vi "String.Remove Invalide Characters from File Name.vi"(8 "error in":errorcluster, 11 "File Name":string) -> (0 "error out":errorcluster, 3 "Valid File Name":string)   [LabVIEW 2018]
panel:
  # "Invalid file name characters for Windows:"
  # "A filename cannot contain any of the following characters:\n  \\ / : * ? \" < > |"
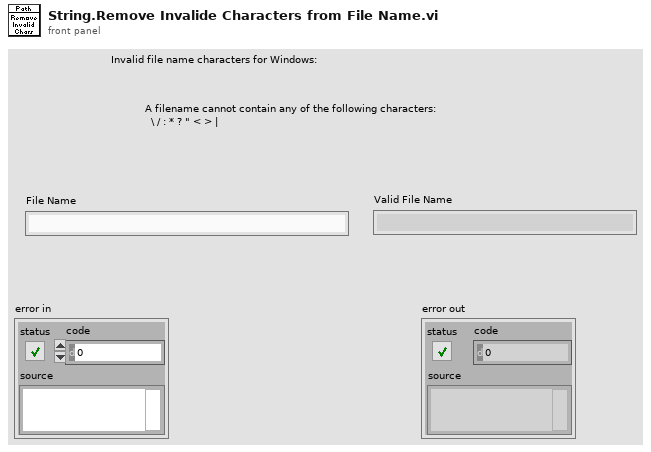
[diagram p1: front panel]
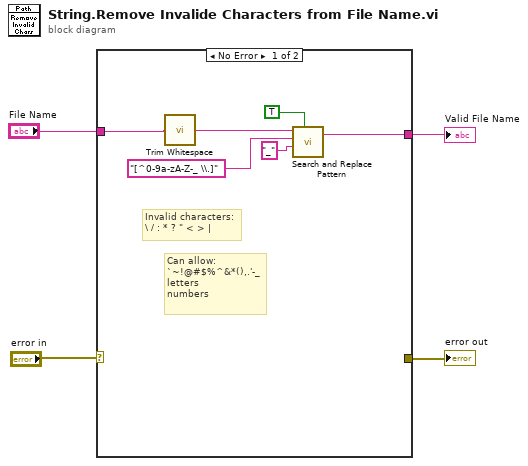
[diagram p0: block diagram]
diagram:
  n1 = case shown="No Error" "error in" {
    selector: "error in" -> [_ w11]
    tunnel: [w7 w12] -> w4
    tunnel: "File Name" -> [w6 w12]
    tunnel: [_ w11] -> w1
    frame No Error {
      # "Can allow:\n`~!@#$%^&*(),.'-_\nletters\nnumbers"
      # "Invalid characters:\n\\ / : * ? \" < > |"
      n2 = call <vilib>:"Trim Whitespace.vi"("string"=w6) -> ("trimmed string"=w5:string)  [unwired: 1 in]
      n3 = call <vilib>:"Search and Replace Pattern.vi"("string"=w5, "regular expression (\"\")"="[^0-9a-zA-Z-_ \\.]" ("regular expression (\"\")"), "replace string (\"\")"="_" ("replace string (\"\")"), "replace all? (F)"=TRUE) -> ("result string"=w7:string)  [unwired: 1 in, 1 out]
    }
    frame Error {
    }
  }
  "Valid File Name" <- w4
  "error out" <- w1
